vi "S2C_ExeLoadTestCheck.vi"(8 "Error In":errorcluster, 11 "FilePath":path) -> (0 "Error Out":errorcluster, 2 "Valid?":bool, 3 "FileRef Out":T1)   [LabVIEW 2015]
doc: "Converts a script line entry into an executable table entry."
uses:
  <vilib>/Utility/config.llb/Config Data RefNum.ctl
  <vilib>/Utility/config.llb/Read Key (String).vi
  <vilib>/Utility/config.llb/NI_LVConfig.lvlib
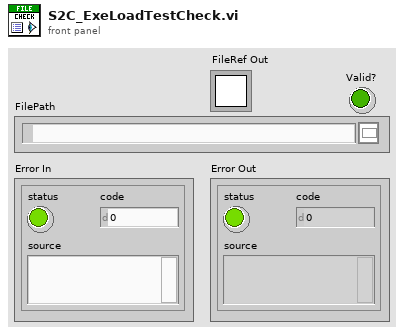
[diagram p1: front panel]
types:
  T1 = typedef "NI_LVConfig.lvlib/Config Data RefNum.ctl" = refnum<k1>
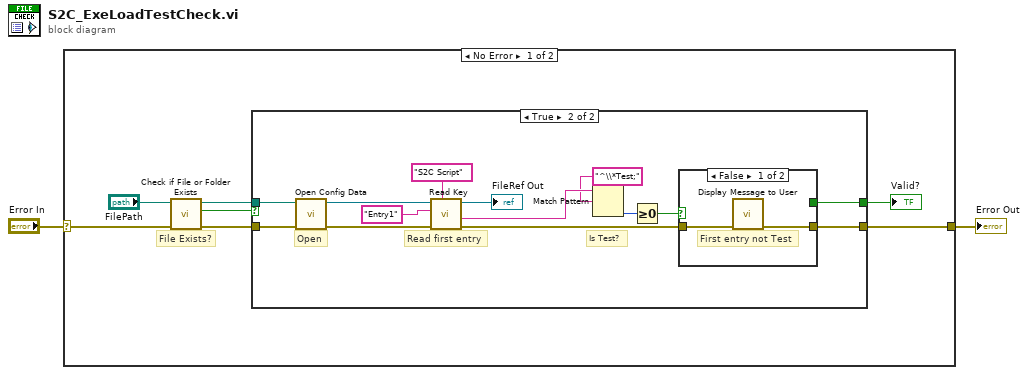
[diagram p0: block diagram]
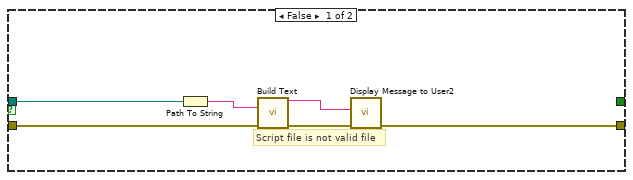
[diagram p2: hidden frame]
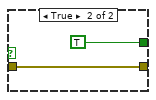
[diagram p3: hidden frame]
diagram:
  n1 = case shown="No Error" "Error In" {
    selector: "Error In" -> [w7 w34]
    tunnel: [w9 w34] -> w1
    frame No Error {
      # "File Exists?"
      n2 = call <vilib>:"Check if File or Folder Exists.vi"("error in (no error)"=w7, "path"="FilePath") -> ("error out"=w5:errorcluster, "file or folder exists?"=w4:bool, "dup path"=w3:path)  [unwired: 7 in]
      n3 = case shown="True" w4 {
        tunnel: [w13 w21] -> w9
        tunnel: [_ w20] -> w8
        tunnel: w5 -> [w15 w16]
        tunnel: w3 -> [w11 w17]
        frame False {
          # "Script file is not valid file"
          n4 = Path To String(path=w11) -> (string=w10:string)
          n5 = call "Build Text"("Script"=w10, "error in (no error)"=w15) -> ("Result"=w12:string, "error out"=w14:errorcluster)  [unwired: 12 in]
          n6 = call "Display Message to User2"("error in (no error)"=w14, "Message"=w12) -> ("error out"=w13:errorcluster)  [unwired: 8 in, 1 out]
        }
        frame True {
          # "Open"
          # "Is Test?"
          # "Read first entry"
          n7 = call <vilib>:"Open Config Data.vi"("error in (no error)"=w16, "configuration file path"=w17) -> ("error out"=w19:errorcluster, "refnum"=w18:T1)  [unwired: 7 in, 1 out]
          n8 = call-poly <vilib>:"Read Key.vi"("section"="S2C Script", "error in (no error)"=w19, "key"="Entry1", "refnum"=w18) -> ("error out"=w22:errorcluster, "value"=w27:string, "refnum out"=→"FileRef Out":T1)  [unwired: 4 in, 1 out]
          n9 = Match Pattern(string=w27, regular expression="^\\*Test;") -> (offset past match=w23:i32)  [unwired: 1 in, 3 out]
          n10 = Greater Or Equal To 0?(x=w23) -> (x >= 0?=w24:bool)
          n11 = case shown="False" w24 {
            tunnel: w22 -> [w31 w33]
            tunnel: [w30 w33] -> w21
            tunnel: [_ TRUE] -> w20
            frame False {
              # "First entry not Test"
              n12 = call "Display Message to User"("error in (no error)"=w31) -> ("error out"=w30:errorcluster)  [unwired: 9 in, 1 out]
            }
            frame True {
            }
          }
        }
      }
      "Valid?" <- w8
    }
    frame Error {
    }
  }
  "Error Out" <- w1
